vi "Set Address.vi"(10 "address":u64 format="%016x", 11 "Pointer in":refnum<class "Pointer.lvclass">) -> (3 "Pointer out":refnum<class "Pointer.lvclass">)   [LabVIEW 2017, in "Memory Manager.lvlib" / "Pointer.lvclass"]
uses:
  Pointer.lvclass
  Pointer.lvclass/Pointer.ctl
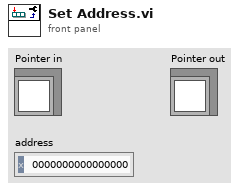
[diagram p1: front panel]
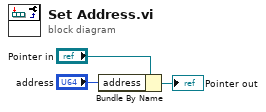
[diagram p0: block diagram]
diagram:
  n1 = Bundle By Name(cluster="Pointer in", "address"="address") -> (→"Pointer out":refnum<class "Pointer.lvclass">)
